vi "TestConfig.vi"() -> ()   [LabVIEW 2014]
uses:
  Config.lvclass
panel:
  in  "btnSettings":bool
  in  "btnStop":bool
  in  "AppData File Path":string="PMUCal\\PMUCal.ini"
  out "ErrorArray out":errorcluster[](array[cluster])
  in  "ErrorArray in":errorcluster[](array[cluster])
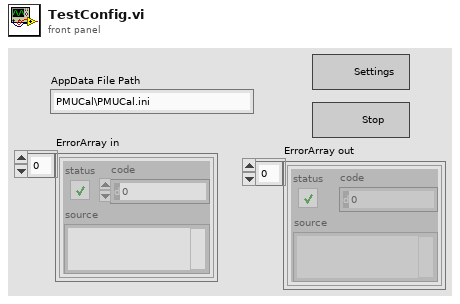
[diagram p1: front panel]
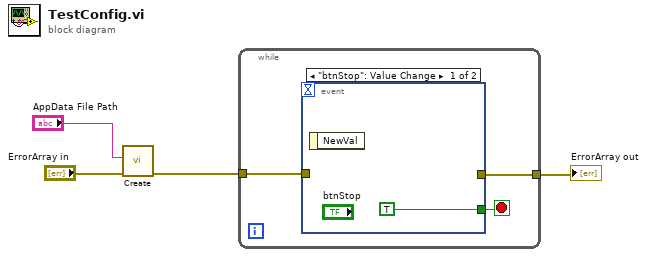
[diagram p0: block diagram]
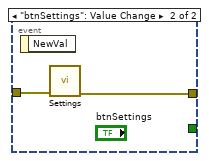
[diagram p2: hidden frame]
diagram:
  n1 = call "Create.vi"("ErrorArray"="ErrorArray in", "name or relative path"="AppData File Path") -> ("ErrorArray"=w2:errorcluster[])  [unwired: 8 in, 1 out]
  n2 = while {
    tunnel: w2 -> [w7]
    tunnel: [w5] -> w1
    stop <- w6 stop-if-true
    n3 = event shown="[0] \"btnStop\": Value Change" {
      selector: _ -> [_ _]
      dyn-events: _ -> [_ _]
      timeout: _ -> [_ _]
      tunnel: w7 -> [_ w10]
      tunnel: [TRUE _] -> w6
      tunnel: [_ w9] -> w5
      event "btnStop": Value Change {
        n4 = event-data() -> ()  [unwired: 1 in, 1 out]
      }
      event "btnSettings": Value Change {
        n5 = event-data() -> ()  [unwired: 1 in, 1 out]
        n6 = call "Settings.vi"("ErrorArray"=w10) -> ("ErrorArray"=w9:errorcluster[])  [unwired: 10 in]
      }
    }
  }
  "ErrorArray out" <- w1
